vi "Put tote down.vi"(8 "rt fifo in out":refnum<k33>) -> (0 "rt fifo out":refnum<k33>)   [LabVIEW 2014]
uses:
  TeleopCmd.ctl
  CmdFlag.ctl
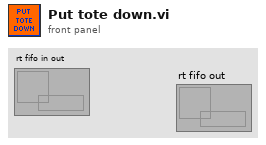
[diagram p1: front panel]
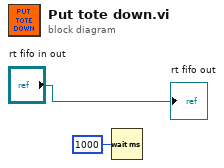
[diagram p0: block diagram]
diagram:
  n1 = Wait (ms)(milliseconds to wait=u32 1000) -> ()  [unwired: 1 out]
  "rt fifo out" <- "rt fifo in out"
